vi "Instr Common Configure.vi"(0 "RFmx Handle In":refnum<k21>, 1 "Selector String":string, 5 "Common Configuration":T1 {"Auto LO Shared" items=["False", "True"]}, 11 "error in (no error)":errorcluster) -> (4 "RFmx Handle Out":refnum<k21>, 15 "error out":errorcluster)   [LabVIEW 2016, in "RFmxInstr.lvlib"]
uses:
  RFmxInstr.lvlib
  Typedefs/Instr Common Configuration.ctl
  <resource>/objmgr/RFmxInstr.rc
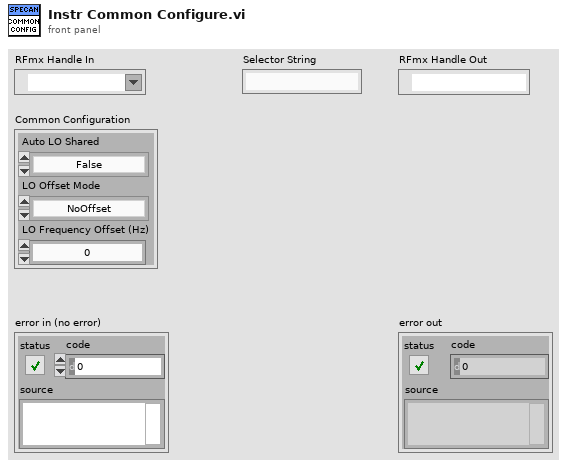
[diagram p1: front panel]
types:
  T1 = typedef "RFmxInstr.lvlib/Instr Common Configuration.ctl" = cluster{"Auto LO Shared":i32, "LO Offset Mode":enum16{"NoOffset", "Automatic", "UserDefined"}, "LO Frequency Offset (Hz)":dbl}
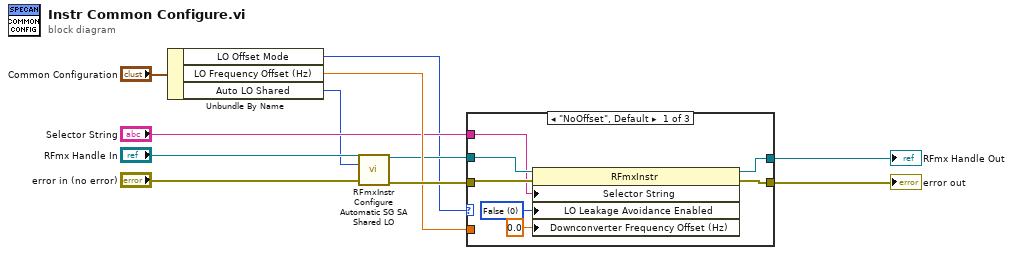
[diagram p0: block diagram]
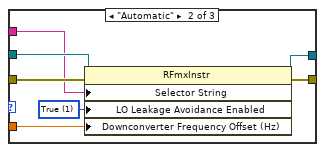
[diagram p2: hidden frame]
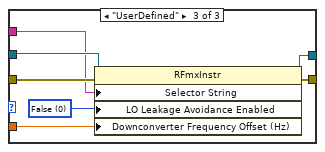
[diagram p3: hidden frame]
diagram:
  n1 = Unbundle By Name("Common Configuration") -> ("LO Offset Mode"=w1:enum16{"NoOffset", "Automatic", "UserDefined"}, "LO Frequency Offset (Hz)"=w7:dbl, "Auto LO Shared"=w2:i32)
  n2 = call <vilib>:"RFmxInstr Configure Automatic SG SA Shared LO.vi"("Instrument Handle In"="RFmx Handle In", "Automatic SG SA Shared LO"=w2, "error in (no error)"="error in (no error)") -> ("Instrument Handle Out"=w6:refnum<k21>, "error out"=w9:errorcluster)  [unwired: 11 in]
  n3 = case shown="\"NoOffset\", Default" w1 {
    tunnel: w9 -> [w17 w25 w30]
    tunnel: [w18 w24 w29] -> w8
    tunnel: w7 -> [_ w20 w26]
    tunnel: w6 -> [w16 w23 w32]
    tunnel: [w15 w22 w31] -> w5
    tunnel: "Selector String" -> [w14 w21 w28]
    frame "NoOffset", Default {
      w12 = 0 items=["False", "True"] ("LO Leakage Avoidance Enabled")
      n4 = property class="RFmxInstr"(reference=w16, error in=w17, "Selector String"=w14, "LO Leakage Avoidance Enabled"=w12, "Downconverter Frequency Offset (Hz)"=0.0) -> (reference out=w15:refnum<k21>, error out=w18:errorcluster)
    }
    frame "Automatic" {
      w19 = 1 items=["False", "True"] ("LO Leakage Avoidance Enabled")
      n5 = property class="RFmxInstr"(reference=w23, error in=w25, "Selector String"=w21, "LO Leakage Avoidance Enabled"=w19, "Downconverter Frequency Offset (Hz)"=w20) -> (reference out=w22:refnum<k21>, error out=w24:errorcluster)
    }
    frame "UserDefined" {
      w27 = 0 items=["False", "True"] ("LO Leakage Avoidance Enabled")
      n6 = property class="RFmxInstr"(reference=w32, error in=w30, "Selector String"=w28, "LO Leakage Avoidance Enabled"=w27, "Downconverter Frequency Offset (Hz)"=w26) -> (reference out=w31:refnum<k21>, error out=w29:errorcluster)
    }
  }
  "error out" <- w8
  "RFmx Handle Out" <- w5
